vi "Ticker Example.vi"   [LabVIEW 2014]
uses:
  QwaveSys_ESP8266/QwaveSys_ESP8266.lvlib
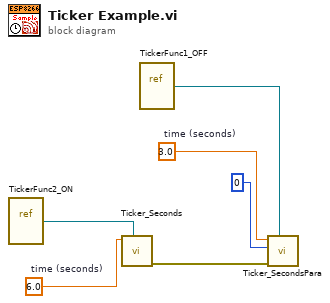
[diagram p0: block diagram]
diagram:
  w2 = 3.0  # time (seconds)
  w3 = 6.0  # time (seconds)
  n1 = vi-ref "TickerFunc2_ON.vi"() -> (w5:refnum<vi>)
  n2 = call "Ticker_Seconds.vi"("VI Refnum"=w5, "time (seconds)"=w3) -> ("error out"=w6:errorcluster)  [unwired: 9 in]
  n3 = vi-ref "TickerFunc1_OFF.vi"() -> (w4:refnum<vi>)
  n4 = call "Ticker_SecondsPara.vi"("VI Refnum"=w4, "error in (no error)"=w6, "data"=u32 0, "time (seconds)"=w2) -> ()  [unwired: 7 in, 1 out]
